vi "Tester.vi"() -> ()   [LabVIEW 2011]
uses:
  <vilib>/Rock Robotics/SystemInterfaces/DIO/FPGA_DIOChannel.ctl
  <vilib>/Rock Robotics/SystemInterfaces/Typedef/FPGA_TypedefDigitalModule.ctl
  <vilib>/Rock Robotics/SystemInterfaces/AI/FPGA_AIChannel.ctl
  <vilib>/Rock Robotics/SystemInterfaces/Typedef/FPGA_TypedefAnalogModule.ctl
  <vilib>/Rock Robotics/SystemInterfaces/DIO/FPGA_DIOPWMChannel.ctl
  <vilib>/Rock Robotics/SystemInterfaces/DIO/FPGA_DIORelayChannel.ctl
  <vilib>/Rock Robotics/WPI/Solenoid/WPI_SolenoidChannel.ctl
  <vilib>/Rock Robotics/SystemInterfaces/Typedef/FPGA_TypedefSolenoidModule.ctl
  <vilib>/Rock Robotics/WPI/Joystick/WPI_JoystickDeviceEnum.ctl
  <vilib>/Rock Robotics/WPI/Solenoid/WPI_SolenoidValue.ctl
  <vilib>/Rock Robotics/WPI/Relay/WPI_RelayValue.ctl
  <vilib>/Rock Robotics/WPI/MotorControl/WPI_MotorControlOpen Jaguar.vi
  <vilib>/Rock Robotics/WPI/Solenoid/WPI_SolenoidOpenSingle.vi
  <vilib>/Rock Robotics/WPI/Solenoid/Deprecated/WPI_SolenoidGetBool.vi
  <vilib>/Rock Robotics/WPI/Solenoid/WPI_SolenoidSetEnum.vi
panel:
  out "Boolean 12":bool
  out "Boolean 11":bool
  out "Boolean 10":bool
  out "Boolean 9":bool
  out "Boolean 8":bool
  out "Boolean 7":bool
  out "Boolean 6":bool
  out "Boolean 5":bool
  out "Boolean 4":bool
  out "Boolean 3":bool
  out "Boolean 2":bool
  out "Boolean":bool
  out "Axis 6":u8
  out "Axis 5":u8
  out "Axis 4":u8
  out "Axis 3 (Throttle)":u8
  out "Axis 2 (Y)":u8
  out "Axis 1 (X)":u8
  in  "Solenoid 8":bool
  in  "Solenoid 7":bool
  in  "Solenoid 6":bool
  in  "Solenoid 5":bool
  in  "Solenoid 4":bool
  in  "Solenoid 3":bool
  in  "Solenoid 2":bool
  in  "Solenoid 1":bool
  in  "Relay 8":bool
  in  "Relay 7":bool
  in  "Relay 6":bool
  in  "Relay 5":bool
  in  "Relay 4":bool
  in  "Relay 3":bool
  in  "Relay 2":bool
  in  "Relay 1":bool
  in  "PWM 10":dbl(knob) scale=-1.0..1.0
  in  "PWM 9":dbl(knob) scale=-1.0..1.0
  in  "PWM 8":dbl(knob) scale=-1.0..1.0
  in  "PWM 7":dbl(knob) scale=-1.0..1.0
  in  "PWM 6":dbl(knob) scale=-1.0..1.0
  in  "PWM 5":dbl(knob) scale=-1.0..1.0
  in  "PWM 4":dbl(knob) scale=-1.0..1.0
  in  "PWM 3":dbl(knob) scale=-1.0..1.0
  in  "PWM 2":dbl(knob) scale=-1.0..1.0
  in  "PWM 1":dbl(knob) scale=-1.0..1.0
  out "Analog 8":dbl
  out "Analog 7":dbl
  out "Analog 6":dbl
  out "Analog 5":dbl
  out "Analog 4":dbl
  out "Analog 3":dbl
  out "Analog 2":dbl
  out "Analog 1":dbl
  out "DIO 14":bool
  out "DIO 13":bool
  out "DIO 12":bool
  out "DIO 11":bool
  out "DIO 10":bool
  out "DIO 9":bool
  out "DIO 8":bool
  out "DIO 7":bool
  out "DIO 6":bool
  out "DIO 5":bool
  out "DIO 4":bool
  out "DIO 3":bool
  out "DIO 2":bool
  out "DIO 1":bool
  # "DIO"
  # "PWM Channels"
  # "Relays"
  # "Solenoids"
  # "Analog"
  # "Joystick"
  # "Buttons"
  # "Axis"
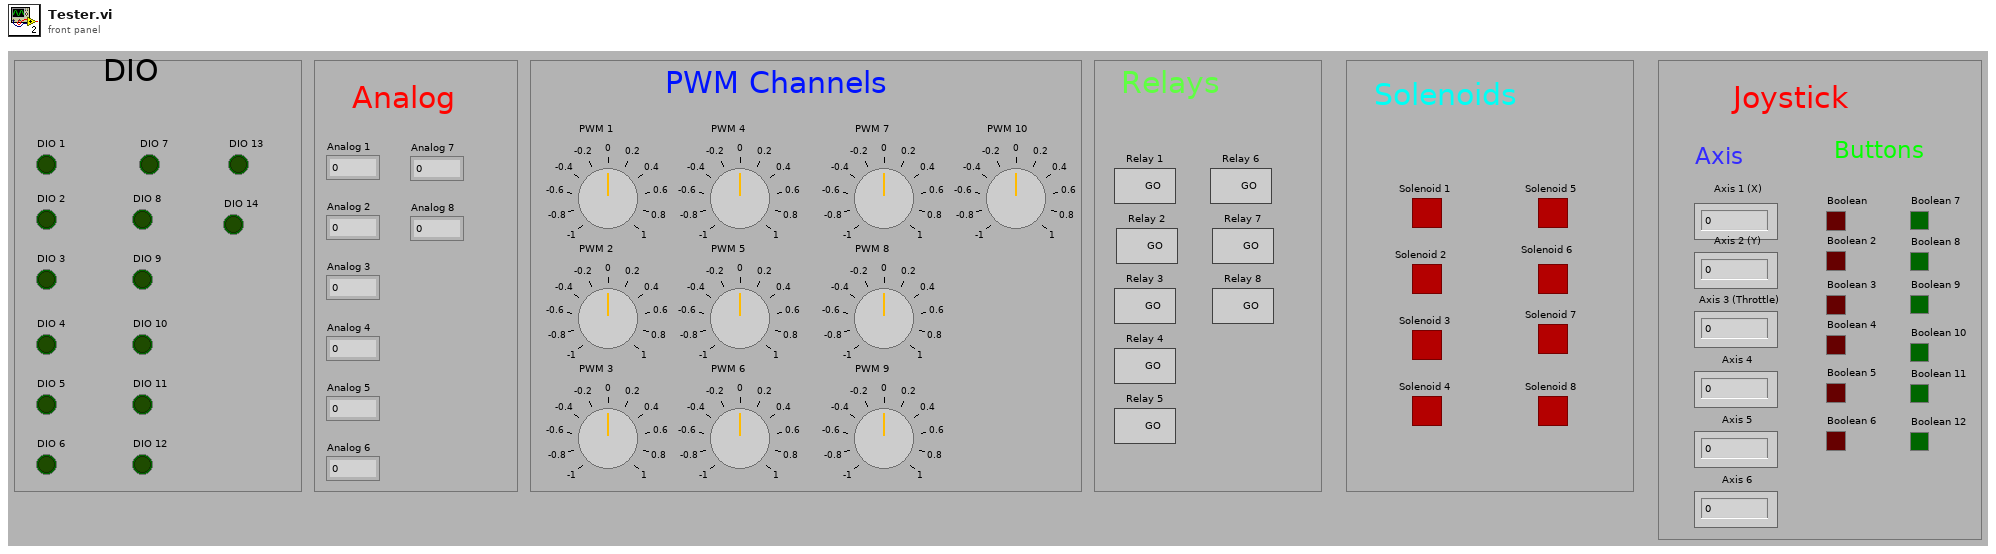
[diagram p1: front panel]
types:
  T1 = typedef "WPI_JoystickDeviceEnum.ctl" = enum16{"USB 1", "USB 2", "USB 3", "USB 4", "Kinect 1", "Kinect 2"}
  T2 = typedef "WPI_SolenoidChannel.ctl" = enum8{"Solenoid 1", "Solenoid 2", "Solenoid 3", "Solenoid 4", "Solenoid 5", "Solenoid 6", "Solenoid 7", "Solenoid 8", "Invalid"}
  T3 = typedef "FPGA_TypedefSolenoidModule.ctl" = enum16{"Solenoid Module 1", "Solenoid Module 2"}
  T4 = typedef "FPGA_DIORelayChannel.ctl" = enum8{"Relay 1", "Relay 2", "Relay 3", "Relay 4", "Relay 5", "Relay 6", "Relay 7", "Relay 8", "Invalid"}
  T5 = typedef "FPGA_TypedefDigitalModule.ctl" = enum16{"Digital Module 1", "Digital Module 2"}
  T6 = typedef "FPGA_DIOPWMChannel.ctl" = enum8{"PWM 1", "PWM 2", "PWM 3", "PWM 4", "PWM 5", "PWM 6", "PWM 7", "PWM 8", "PWM 9", "PWM 10", "Invalid"}
  T7 = typedef "FPGA_AIChannel.ctl" = enum8{"AI 1", "AI 2", "AI 3", "AI 4", "AI 5", "AI 6", "AI 7", "AI 8", "Invalid"}
  T8 = typedef "FPGA_TypedefAnalogModule.ctl" = enum16{"Analog Module 1", "Analog Module 2"}
  T9 = typedef "FPGA_DIOChannel.ctl" = enum8{"DIO 1", "DIO 2", "DIO 3", "DIO 4", "DIO 5", "DIO 6", "DIO 7", "DIO 8", "DIO 9", "DIO 10", "DIO 11", "DIO 12", "DIO 13", "DIO 14", "Invalid"}
  T10 = typedef "WPI_MotorControlDeviceRef.ctl" = cluster{"DeviceStatus":errorcluster, "Type":enum16{"PWM", "CAN"}, "PWM":cluster{"Digital Module":T5, "PWM Channel":T6, "DeadBand":T11}, "CAN":cluster{"Device Number":u8, "Control Mode":T12, "Semaphore":T13, "Max Vout":dbl}, "Invert":bool, "TransformRef":T14, "InvTransformRef":T14}
  T11 = typedef "WPI_PWMDeadband.ctl" = cluster{"Name":string, "maxPositivePwm":i32, "minPositivePwm":i32, "centerPwm":i32, "maxNegativePwm":i32, "minNegativePwm":i32, "angularRange":u16}
  T12 = typedef "WPI_CANJaguar_ControlMode.ctl" = enum8{"Percent VBus", "Current", "Speed", "Position", "Voltage"}
  T13 = typedef "Semaphore RefNum" = refnum<k1>
  T14 = typedef "WPI_PWMTransform_ConPane.ctl" = refnum<vi>
  T15 = typedef "WPI_SolenoidDevRef.ctl" = cluster{"DevStatus":errorcluster, "Solenoid Module":T3, "Forward Solenoid Channel":T2, "Reverse Solenoid Channel":T2}
  T16 = typedef "WPI_DigitalInputDevRef.ctl" = cluster{"DevStatus":errorcluster, "DIO Channel":T9, "Digital Module":T5}
  T17 = typedef "WPI_AnalogChannelDevRef.ctl" = cluster{"DevStatus":errorcluster, "Analog Module":T8, "Analog Channel":T7}
  T18 = typedef "WPI_RelayDevRef.ctl" = cluster{"DevStatus":errorcluster, "Relay Channel":T4, "Digital Module":T5, "Relay Direction":T19}
  T19 = typedef "WPI_RelayDirection.ctl" = enum16{"Both directions", "Forward only", "Reverse only"}
  T20 = typedef "WPI_JoystickDevRef.ctl" = cluster{"Device":T1}
  T21 = typedef "WPI_SolenoidValue.ctl" = enum16{"Off", "On", "Forward", "Reverse"}
  T22 = typedef "WPI_RelayValue.ctl" = enum16{"Off", "On", "Forward", "Reverse"}
  T23 = typedef "WPI_JoystickButtonState.ctl" = cluster{"Button 1":bool, "Button 2":bool, "Button 3":bool, "Button 4":bool, "Button 5":bool, "Button 6":bool, "Button 7":bool, "Button 8":bool, "Button 9":bool, "Button 10":bool, "Button 11":bool, "Button 12":bool}
  T24 = cluster{"axis 1 (x)":dbl, "axis 2 (y)":dbl, "axis 3 (throttle)":dbl, "axis 4":dbl, "axis 5":dbl, "axis 6":dbl}
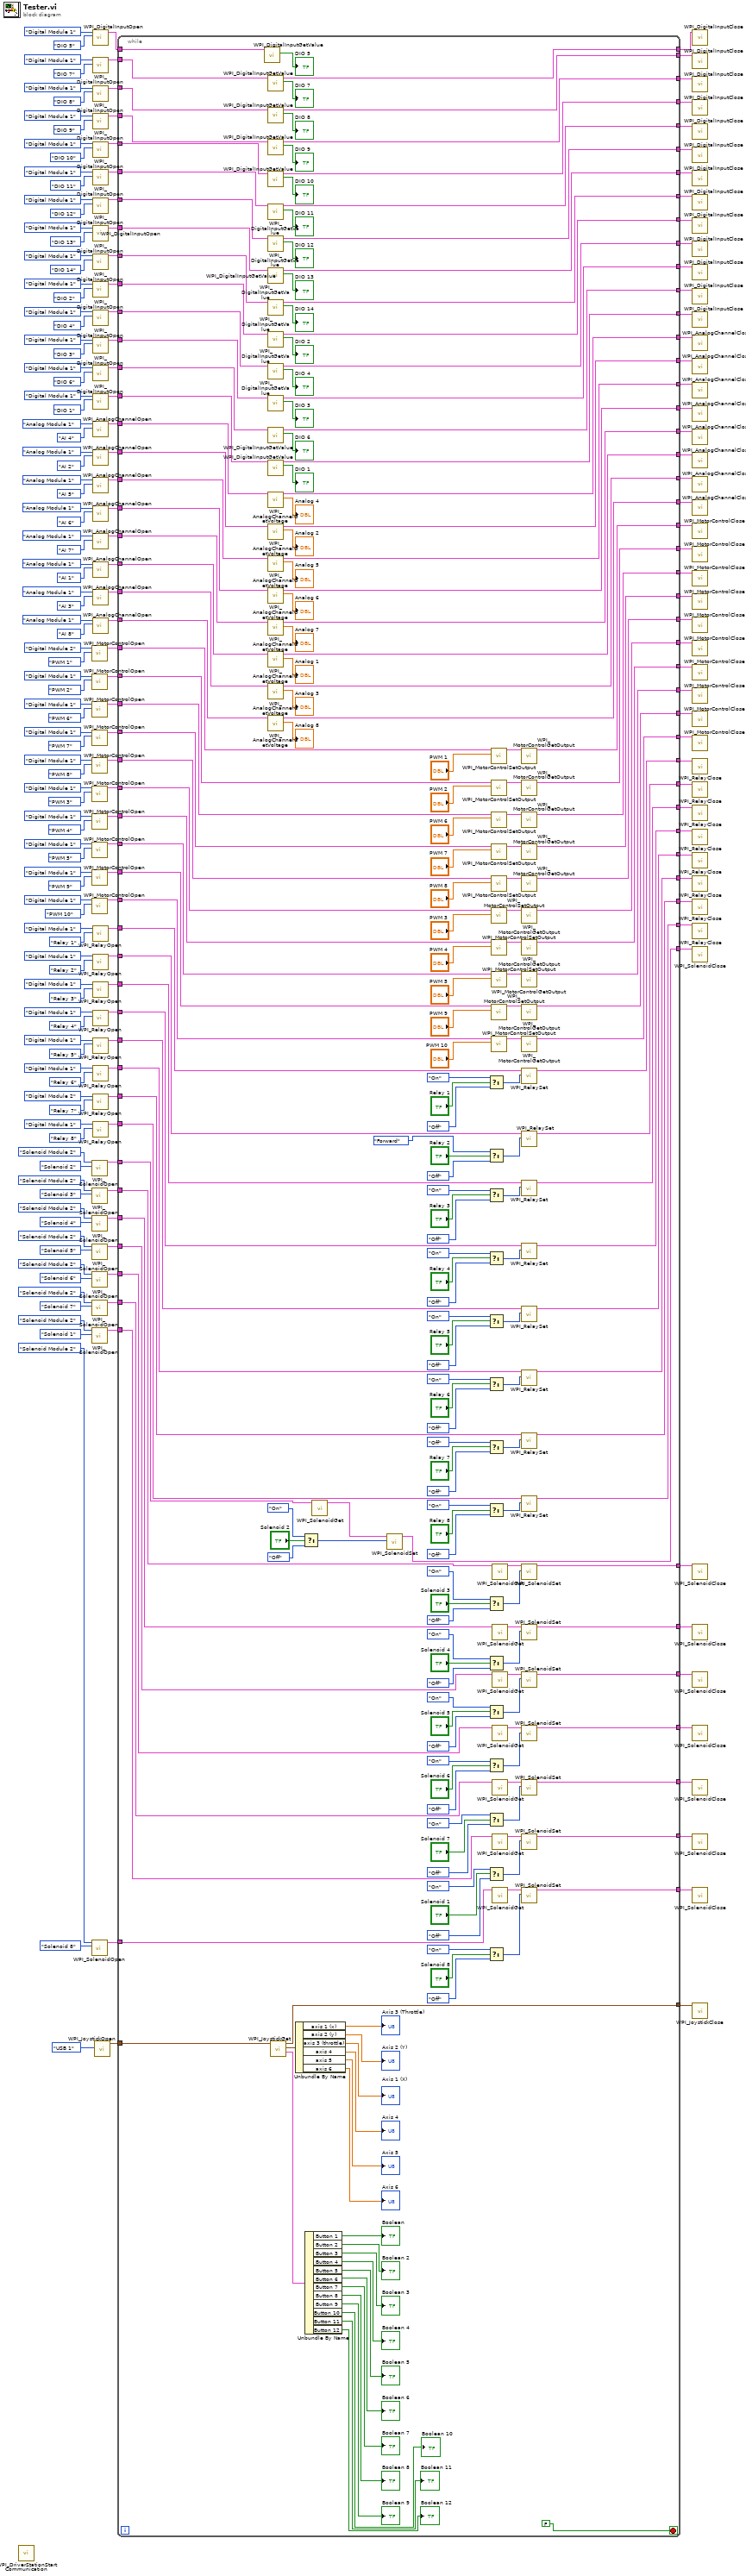
[diagram p0: block diagram]
diagram:
  n1 = call <vilib>:"WPI_DriverStationStart Communication.vi"() -> ()  [unwired: 1 in, 11 out]
  n2 = call-poly <vilib>:"WPI_MotorControlOpen.vi"("PWM Channel"=FPGA_DIOPWMChannel."PWM 1", "Digital Module (Module 1)"=FPGA_TypedefDigitalModule."Digital Module 2" ("DIO Module (Slot 4)")) -> ("MotorControlDeviceRef"=w128:T10)  [unwired: 5 in, 4 out]
  n3 = call-poly <vilib>:"WPI_MotorControlOpen.vi"("PWM Channel"=FPGA_DIOPWMChannel."PWM 2", "Digital Module (Module 1)"=FPGA_TypedefDigitalModule."Digital Module 1" ("DIO Module (Slot 4)")) -> ("MotorControlDeviceRef"=w120:T10)  [unwired: 5 in, 4 out]
  n4 = call-poly <vilib>:"WPI_MotorControlOpen.vi"("PWM Channel"=FPGA_DIOPWMChannel."PWM 6", "Digital Module (Module 1)"=FPGA_TypedefDigitalModule."Digital Module 1" ("DIO Module (Slot 4)")) -> ("MotorControlDeviceRef"=w119:T10)  [unwired: 5 in, 4 out]
  n5 = call-poly <vilib>:"WPI_MotorControlOpen.vi"("PWM Channel"=FPGA_DIOPWMChannel."PWM 7", "Digital Module (Module 1)"=FPGA_TypedefDigitalModule."Digital Module 1" ("DIO Module (Slot 4)")) -> ("MotorControlDeviceRef"=w116:T10)  [unwired: 5 in, 4 out]
  n6 = call-poly <vilib>:"WPI_MotorControlOpen.vi"("PWM Channel"=FPGA_DIOPWMChannel."PWM 8", "Digital Module (Module 1)"=FPGA_TypedefDigitalModule."Digital Module 1" ("DIO Module (Slot 4)")) -> ("MotorControlDeviceRef"=w113:T10)  [unwired: 5 in, 4 out]
  n7 = call-poly <vilib>:"WPI_MotorControlOpen.vi"("PWM Channel"=FPGA_DIOPWMChannel."PWM 3", "Digital Module (Module 1)"=FPGA_TypedefDigitalModule."Digital Module 1" ("DIO Module (Slot 4)")) -> ("MotorControlDeviceRef"=w110:T10)  [unwired: 5 in, 4 out]
  n8 = call-poly <vilib>:"WPI_MotorControlOpen.vi"("PWM Channel"=FPGA_DIOPWMChannel."PWM 4", "Digital Module (Module 1)"=FPGA_TypedefDigitalModule."Digital Module 1" ("DIO Module (Slot 4)")) -> ("MotorControlDeviceRef"=w107:T10)  [unwired: 5 in, 4 out]
  n9 = call-poly <vilib>:"WPI_MotorControlOpen.vi"("PWM Channel"=FPGA_DIOPWMChannel."PWM 5", "Digital Module (Module 1)"=FPGA_TypedefDigitalModule."Digital Module 1" ("DIO Module (Slot 4)")) -> ("MotorControlDeviceRef"=w104:T10)  [unwired: 5 in, 4 out]
  n10 = call-poly <vilib>:"WPI_MotorControlOpen.vi"("PWM Channel"=FPGA_DIOPWMChannel."PWM 9", "Digital Module (Module 1)"=FPGA_TypedefDigitalModule."Digital Module 1" ("DIO Module (Slot 4)")) -> ("MotorControlDeviceRef"=w96:T10)  [unwired: 5 in, 4 out]
  n11 = call-poly <vilib>:"WPI_MotorControlOpen.vi"("PWM Channel"=FPGA_DIOPWMChannel."PWM 10", "Digital Module (Module 1)"=FPGA_TypedefDigitalModule."Digital Module 1" ("DIO Module (Slot 4)")) -> ("MotorControlDeviceRef"=w91:T10)  [unwired: 5 in, 4 out]
  n12 = call-poly <vilib>:"WPI_SolenoidOpen.vi"("Solenoid Channel"=WPI_SolenoidChannel."Solenoid 2", "Solenoid Module (Module 1)"=FPGA_TypedefSolenoidModule."Solenoid Module 2") -> ("SolenoidDevRef"=w61:T15)  [unwired: 8 in, 1 out]
  n13 = call-poly <vilib>:"WPI_SolenoidOpen.vi"("Solenoid Channel"=WPI_SolenoidChannel."Solenoid 3", "Solenoid Module (Module 1)"=FPGA_TypedefSolenoidModule."Solenoid Module 2") -> ("SolenoidDevRef"=w60:T15)  [unwired: 8 in, 1 out]
  n14 = call-poly <vilib>:"WPI_SolenoidOpen.vi"("Solenoid Channel"=WPI_SolenoidChannel."Solenoid 4", "Solenoid Module (Module 1)"=FPGA_TypedefSolenoidModule."Solenoid Module 2") -> ("SolenoidDevRef"=w59:T15)  [unwired: 8 in, 1 out]
  n15 = call-poly <vilib>:"WPI_SolenoidOpen.vi"("Solenoid Channel"=WPI_SolenoidChannel."Solenoid 5", "Solenoid Module (Module 1)"=FPGA_TypedefSolenoidModule."Solenoid Module 2") -> ("SolenoidDevRef"=w58:T15)  [unwired: 8 in, 1 out]
  n16 = call-poly <vilib>:"WPI_SolenoidOpen.vi"("Solenoid Channel"=WPI_SolenoidChannel."Solenoid 6", "Solenoid Module (Module 1)"=FPGA_TypedefSolenoidModule."Solenoid Module 2") -> ("SolenoidDevRef"=w57:T15)  [unwired: 8 in, 1 out]
  n17 = call-poly <vilib>:"WPI_SolenoidOpen.vi"("Solenoid Channel"=WPI_SolenoidChannel."Solenoid 7", "Solenoid Module (Module 1)"=FPGA_TypedefSolenoidModule."Solenoid Module 2") -> ("SolenoidDevRef"=w56:T15)  [unwired: 8 in, 1 out]
  n18 = call-poly <vilib>:"WPI_SolenoidOpen.vi"("Solenoid Channel"=WPI_SolenoidChannel."Solenoid 1", "Solenoid Module (Module 1)"=FPGA_TypedefSolenoidModule."Solenoid Module 2") -> ("SolenoidDevRef"=w55:T15)  [unwired: 8 in, 1 out]
  n19 = call-poly <vilib>:"WPI_SolenoidOpen.vi"("Solenoid Channel"=WPI_SolenoidChannel."Solenoid 8", "Solenoid Module (Module 1)"=FPGA_TypedefSolenoidModule."Solenoid Module 2") -> ("SolenoidDevRef"=w54:T15)  [unwired: 8 in, 1 out]
  n20 = call <vilib>:"WPI_DigitalInputOpen.vi"("DIO Channel"=FPGA_DIOChannel."DIO 5", "Digital Module (Module 1)"=FPGA_TypedefDigitalModule."Digital Module 1" ("DIO Module (Slot 4)")) -> ("DigitalInputDevRef"=w194:T16)  [unwired: 1 in, 8 out]
  n21 = call <vilib>:"WPI_DigitalInputOpen.vi"("DIO Channel"=FPGA_DIOChannel."DIO 7", "Digital Module (Module 1)"=FPGA_TypedefDigitalModule."Digital Module 1" ("DIO Module (Slot 4)")) -> ("DigitalInputDevRef"=w175:T16)  [unwired: 1 in, 8 out]
  n22 = call <vilib>:"WPI_DigitalInputOpen.vi"("DIO Channel"=FPGA_DIOChannel."DIO 8", "Digital Module (Module 1)"=FPGA_TypedefDigitalModule."Digital Module 1" ("DIO Module (Slot 4)")) -> ("DigitalInputDevRef"=w174:T16)  [unwired: 1 in, 8 out]
  n23 = call <vilib>:"WPI_DigitalInputOpen.vi"("DIO Channel"=FPGA_DIOChannel."DIO 9", "Digital Module (Module 1)"=FPGA_TypedefDigitalModule."Digital Module 1" ("DIO Module (Slot 4)")) -> ("DigitalInputDevRef"=w173:T16)  [unwired: 1 in, 8 out]
  n24 = call <vilib>:"WPI_DigitalInputOpen.vi"("DIO Channel"=FPGA_DIOChannel."DIO 10", "Digital Module (Module 1)"=FPGA_TypedefDigitalModule."Digital Module 1" ("DIO Module (Slot 4)")) -> ("DigitalInputDevRef"=w172:T16)  [unwired: 1 in, 8 out]
  n25 = call <vilib>:"WPI_DigitalInputOpen.vi"("DIO Channel"=FPGA_DIOChannel."DIO 11", "Digital Module (Module 1)"=FPGA_TypedefDigitalModule."Digital Module 1" ("DIO Module (Slot 4)")) -> ("DigitalInputDevRef"=w171:T16)  [unwired: 1 in, 8 out]
  n26 = call <vilib>:"WPI_DigitalInputOpen.vi"("DIO Channel"=FPGA_DIOChannel."DIO 12", "Digital Module (Module 1)"=FPGA_TypedefDigitalModule."Digital Module 1" ("DIO Module (Slot 4)")) -> ("DigitalInputDevRef"=w170:T16)  [unwired: 1 in, 8 out]
  n27 = call <vilib>:"WPI_DigitalInputOpen.vi"("DIO Channel"=FPGA_DIOChannel."DIO 13", "Digital Module (Module 1)"=FPGA_TypedefDigitalModule."Digital Module 1" ("DIO Module (Slot 4)")) -> ("DigitalInputDevRef"=w169:T16)  [unwired: 1 in, 8 out]
  n28 = call <vilib>:"WPI_DigitalInputOpen.vi"("DIO Channel"=FPGA_DIOChannel."DIO 14", "Digital Module (Module 1)"=FPGA_TypedefDigitalModule."Digital Module 1" ("DIO Module (Slot 4)")) -> ("DigitalInputDevRef"=w168:T16)  [unwired: 1 in, 8 out]
  n29 = call <vilib>:"WPI_DigitalInputOpen.vi"("DIO Channel"=FPGA_DIOChannel."DIO 2", "Digital Module (Module 1)"=FPGA_TypedefDigitalModule."Digital Module 1" ("DIO Module (Slot 4)")) -> ("DigitalInputDevRef"=w167:T16)  [unwired: 1 in, 8 out]
  n30 = call <vilib>:"WPI_DigitalInputOpen.vi"("DIO Channel"=FPGA_DIOChannel."DIO 4", "Digital Module (Module 1)"=FPGA_TypedefDigitalModule."Digital Module 1" ("DIO Module (Slot 4)")) -> ("DigitalInputDevRef"=w164:T16)  [unwired: 1 in, 8 out]
  n31 = call <vilib>:"WPI_DigitalInputOpen.vi"("DIO Channel"=FPGA_DIOChannel."DIO 3", "Digital Module (Module 1)"=FPGA_TypedefDigitalModule."Digital Module 1" ("DIO Module (Slot 4)")) -> ("DigitalInputDevRef"=w161:T16)  [unwired: 1 in, 8 out]
  n32 = call <vilib>:"WPI_DigitalInputOpen.vi"("DIO Channel"=FPGA_DIOChannel."DIO 6", "Digital Module (Module 1)"=FPGA_TypedefDigitalModule."Digital Module 1" ("DIO Module (Slot 4)")) -> ("DigitalInputDevRef"=w158:T16)  [unwired: 1 in, 8 out]
  n33 = call <vilib>:"WPI_DigitalInputOpen.vi"("DIO Channel"=FPGA_DIOChannel."DIO 1", "Digital Module (Module 1)"=FPGA_TypedefDigitalModule."Digital Module 1" ("DIO Module (Slot 4)")) -> ("DigitalInputDevRef"=w155:T16)  [unwired: 1 in, 8 out]
  n34 = call <vilib>:"WPI_AnalogChannelOpen.vi"("Analog Channel"=FPGA_AIChannel."AI 4", "Analog Module (Module 1)"=FPGA_TypedefAnalogModule."Analog Module 1" ("Analog Module (Slot 1)")) -> ("AIDeviceRef"=w136:T17)  [unwired: 1 in, 8 out]
  n35 = call <vilib>:"WPI_AnalogChannelOpen.vi"("Analog Channel"=FPGA_AIChannel."AI 2", "Analog Module (Module 1)"=FPGA_TypedefAnalogModule."Analog Module 1" ("Analog Module (Slot 1)")) -> ("AIDeviceRef"=w135:T17)  [unwired: 1 in, 8 out]
  n36 = call <vilib>:"WPI_AnalogChannelOpen.vi"("Analog Channel"=FPGA_AIChannel."AI 5", "Analog Module (Module 1)"=FPGA_TypedefAnalogModule."Analog Module 1" ("Analog Module (Slot 1)")) -> ("AIDeviceRef"=w134:T17)  [unwired: 1 in, 8 out]
  n37 = call <vilib>:"WPI_AnalogChannelOpen.vi"("Analog Channel"=FPGA_AIChannel."AI 6", "Analog Module (Module 1)"=FPGA_TypedefAnalogModule."Analog Module 1" ("Analog Module (Slot 1)")) -> ("AIDeviceRef"=w133:T17)  [unwired: 1 in, 8 out]
  n38 = call <vilib>:"WPI_AnalogChannelOpen.vi"("Analog Channel"=FPGA_AIChannel."AI 7", "Analog Module (Module 1)"=FPGA_TypedefAnalogModule."Analog Module 1" ("Analog Module (Slot 1)")) -> ("AIDeviceRef"=w132:T17)  [unwired: 1 in, 8 out]
  n39 = call <vilib>:"WPI_AnalogChannelOpen.vi"("Analog Channel"=FPGA_AIChannel."AI 1", "Analog Module (Module 1)"=FPGA_TypedefAnalogModule."Analog Module 1" ("Analog Module (Slot 1)")) -> ("AIDeviceRef"=w131:T17)  [unwired: 1 in, 8 out]
  n40 = call <vilib>:"WPI_AnalogChannelOpen.vi"("Analog Channel"=FPGA_AIChannel."AI 3", "Analog Module (Module 1)"=FPGA_TypedefAnalogModule."Analog Module 1" ("Analog Module (Slot 1)")) -> ("AIDeviceRef"=w130:T17)  [unwired: 1 in, 8 out]
  n41 = call <vilib>:"WPI_AnalogChannelOpen.vi"("Analog Channel"=FPGA_AIChannel."AI 8", "Analog Module (Module 1)"=FPGA_TypedefAnalogModule."Analog Module 1" ("Analog Module (Slot 1)")) -> ("AIDeviceRef"=w129:T17)  [unwired: 1 in, 8 out]
  n42 = call <vilib>:"WPI_RelayOpen.vi"("Relay Channel"=FPGA_DIORelayChannel."Relay 1", "Digital Module (Module 1)"=FPGA_TypedefDigitalModule."Digital Module 1" ("DIO Module (Slot 4)")) -> ("RelayDevRef"=w86:T18)  [unwired: 2 in, 7 out]
  n43 = call <vilib>:"WPI_RelayOpen.vi"("Relay Channel"=FPGA_DIORelayChannel."Relay 2", "Digital Module (Module 1)"=FPGA_TypedefDigitalModule."Digital Module 1" ("DIO Module (Slot 4)")) -> ("RelayDevRef"=w84:T18)  [unwired: 2 in, 7 out]
  n44 = call <vilib>:"WPI_RelayOpen.vi"("Relay Channel"=FPGA_DIORelayChannel."Relay 3", "Digital Module (Module 1)"=FPGA_TypedefDigitalModule."Digital Module 1" ("DIO Module (Slot 4)")) -> ("RelayDevRef"=w83:T18)  [unwired: 2 in, 7 out]
  n45 = call <vilib>:"WPI_RelayOpen.vi"("Relay Channel"=FPGA_DIORelayChannel."Relay 4", "Digital Module (Module 1)"=FPGA_TypedefDigitalModule."Digital Module 1" ("DIO Module (Slot 4)")) -> ("RelayDevRef"=w82:T18)  [unwired: 2 in, 7 out]
  n46 = call <vilib>:"WPI_RelayOpen.vi"("Relay Channel"=FPGA_DIORelayChannel."Relay 5", "Digital Module (Module 1)"=FPGA_TypedefDigitalModule."Digital Module 1" ("DIO Module (Slot 4)")) -> ("RelayDevRef"=w81:T18)  [unwired: 2 in, 7 out]
  n47 = call <vilib>:"WPI_RelayOpen.vi"("Relay Channel"=FPGA_DIORelayChannel."Relay 6", "Digital Module (Module 1)"=FPGA_TypedefDigitalModule."Digital Module 1" ("DIO Module (Slot 4)")) -> ("RelayDevRef"=w80:T18)  [unwired: 2 in, 7 out]
  n48 = call <vilib>:"WPI_RelayOpen.vi"("Relay Channel"=FPGA_DIORelayChannel."Relay 7", "Digital Module (Module 1)"=FPGA_TypedefDigitalModule."Digital Module 2" ("DIO Module (Slot 4)")) -> ("RelayDevRef"=w79:T18)  [unwired: 2 in, 7 out]
  n49 = call <vilib>:"WPI_RelayOpen.vi"("Relay Channel"=FPGA_DIORelayChannel."Relay 8", "Digital Module (Module 1)"=FPGA_TypedefDigitalModule."Digital Module 1" ("DIO Module (Slot 4)")) -> ("RelayDevRef"=w78:T18)  [unwired: 2 in, 7 out]
  n50 = call <vilib>:"WPI_JoystickOpen.vi"("JoystickDevice"=WPI_JoystickDeviceEnum."USB 1") -> ("JoystickDevRef"=w3:T20)  [unwired: 10 in]
  n51 = while {
    tunnel: w194 -> [w425]
    tunnel: w175 -> [w424]
    tunnel: w174 -> [w423]
    tunnel: w173 -> [w422]
    tunnel: w172 -> [w421]
    tunnel: w171 -> [w420]
    tunnel: w170 -> [w419]
    tunnel: w169 -> [w418]
    tunnel: w168 -> [w417]
    tunnel: w167 -> [w416]
    tunnel: w164 -> [w415]
    tunnel: w161 -> [w414]
    tunnel: w158 -> [w413]
    tunnel: w155 -> [w412]
    tunnel: w136 -> [w411]
    tunnel: w135 -> [w410]
    tunnel: w134 -> [w409]
    tunnel: w133 -> [w408]
    tunnel: w132 -> [w407]
    tunnel: w131 -> [w406]
    tunnel: w130 -> [w405]
    tunnel: w129 -> [w404]
    tunnel: w128 -> [w381]
    tunnel: [w379] -> w127
    tunnel: w120 -> [w371]
    tunnel: w119 -> [w370]
    tunnel: w116 -> [w369]
    tunnel: w113 -> [w368]
    tunnel: w110 -> [w367]
    tunnel: w107 -> [w366]
    tunnel: w104 -> [w365]
    tunnel: [w364] -> w103
    tunnel: [w363] -> w102
    tunnel: [w362] -> w101
    tunnel: [w361] -> w100
    tunnel: [w360] -> w99
    tunnel: [w359] -> w98
    tunnel: [w358] -> w97
    tunnel: w96 -> [w347]
    tunnel: w91 -> [w345]
    tunnel: [w343] -> w90
    tunnel: [w342] -> w89
    tunnel: w86 -> [w341]
    tunnel: [w340] -> w85
    tunnel: w84 -> [w339]
    tunnel: w83 -> [w338]
    tunnel: w82 -> [w337]
    tunnel: w81 -> [w336]
    tunnel: w80 -> [w335]
    tunnel: w79 -> [w334]
    tunnel: w78 -> [w333]
    tunnel: w61 -> [w332]
    tunnel: w60 -> [w331]
    tunnel: w59 -> [w330]
    tunnel: w58 -> [w329]
    tunnel: w57 -> [w328]
    tunnel: w56 -> [w327]
    tunnel: w55 -> [w326]
    tunnel: w54 -> [w325]
    tunnel: [w296] -> w53
    tunnel: [w295] -> w52
    tunnel: [w294] -> w51
    tunnel: [w293] -> w50
    tunnel: [w292] -> w49
    tunnel: [w291] -> w48
    tunnel: [w290] -> w47
    tunnel: [w289] -> w46
    tunnel: [w288] -> w45
    tunnel: [w287] -> w44
    tunnel: [w286] -> w43
    tunnel: [w285] -> w42
    tunnel: [w284] -> w41
    tunnel: [w283] -> w40
    tunnel: [w278] -> w39
    tunnel: [w269] -> w38
    tunnel: [w268] -> w37
    tunnel: [w267] -> w36
    tunnel: [w266] -> w35
    tunnel: [w265] -> w34
    tunnel: [w264] -> w33
    tunnel: [w263] -> w32
    tunnel: [w262] -> w31
    tunnel: [w261] -> w30
    tunnel: [w260] -> w29
    tunnel: [w259] -> w28
    tunnel: [w258] -> w27
    tunnel: [w257] -> w26
    tunnel: [w256] -> w25
    tunnel: [w255] -> w24
    tunnel: [w254] -> w23
    tunnel: [w253] -> w22
    tunnel: [w252] -> w21
    tunnel: [w251] -> w20
    tunnel: [w250] -> w19
    tunnel: [w249] -> w18
    tunnel: w3 -> [w216]
    tunnel: [w215] -> w2
    stop <- FALSE stop-if-true
    n52 = call <vilib>:"WPI_DigitalInputGetValue.vi"("DigitalInputDevRef"=w425) -> ("Value"=→"DIO 5":bool)  [unwired: 1 in, 9 out]
    n53 = call <vilib>:"WPI_DigitalInputGetValue.vi"("DigitalInputDevRef"=w424) -> ("Value"=→"DIO 7":bool, "DigitalInputDevRef"=w258:T16)  [unwired: 1 in, 8 out]
    n54 = call <vilib>:"WPI_DigitalInputGetValue.vi"("DigitalInputDevRef"=w423) -> ("Value"=→"DIO 8":bool, "DigitalInputDevRef"=w259:T16)  [unwired: 1 in, 8 out]
    n55 = call <vilib>:"WPI_DigitalInputGetValue.vi"("DigitalInputDevRef"=w422) -> ("Value"=→"DIO 9":bool, "DigitalInputDevRef"=w260:T16)  [unwired: 1 in, 8 out]
    n56 = call <vilib>:"WPI_DigitalInputGetValue.vi"("DigitalInputDevRef"=w421) -> ("Value"=→"DIO 10":bool, "DigitalInputDevRef"=w263:T16)  [unwired: 1 in, 8 out]
    n57 = call <vilib>:"WPI_DigitalInputGetValue.vi"("DigitalInputDevRef"=w420) -> ("Value"=→"DIO 11":bool, "DigitalInputDevRef"=w261:T16)  [unwired: 1 in, 8 out]
    n58 = call <vilib>:"WPI_DigitalInputGetValue.vi"("DigitalInputDevRef"=w419) -> ("Value"=→"DIO 12":bool, "DigitalInputDevRef"=w262:T16)  [unwired: 1 in, 8 out]
    n59 = call <vilib>:"WPI_DigitalInputGetValue.vi"("DigitalInputDevRef"=w418) -> ("Value"=→"DIO 13":bool, "DigitalInputDevRef"=w257:T16)  [unwired: 1 in, 8 out]
    n60 = call <vilib>:"WPI_DigitalInputGetValue.vi"("DigitalInputDevRef"=w417) -> ("Value"=→"DIO 14":bool, "DigitalInputDevRef"=w264:T16)  [unwired: 1 in, 8 out]
    n61 = call <vilib>:"WPI_DigitalInputGetValue.vi"("DigitalInputDevRef"=w416) -> ("Value"=→"DIO 2":bool, "DigitalInputDevRef"=w265:T16)  [unwired: 1 in, 8 out]
    n62 = call <vilib>:"WPI_DigitalInputGetValue.vi"("DigitalInputDevRef"=w415) -> ("Value"=→"DIO 4":bool, "DigitalInputDevRef"=w266:T16)  [unwired: 1 in, 8 out]
    n63 = call <vilib>:"WPI_DigitalInputGetValue.vi"("DigitalInputDevRef"=w414) -> ("Value"=→"DIO 3":bool, "DigitalInputDevRef"=w267:T16)  [unwired: 1 in, 8 out]
    n64 = call <vilib>:"WPI_DigitalInputGetValue.vi"("DigitalInputDevRef"=w413) -> ("Value"=→"DIO 6":bool, "DigitalInputDevRef"=w268:T16)  [unwired: 1 in, 8 out]
    n65 = call <vilib>:"WPI_DigitalInputGetValue.vi"("DigitalInputDevRef"=w412) -> ("Value"=→"DIO 1":bool, "DigitalInputDevRef"=w269:T16)  [unwired: 1 in, 8 out]
    n66 = call <vilib>:"WPI_AnalogChannelGetVoltage.vi"("AIDeviceRef"=w411) -> ("Voltage"=→"Analog 4":dbl, "AIDeviceRef"=w256:T17)  [unwired: 1 in, 8 out]
    n67 = call <vilib>:"WPI_AnalogChannelGetVoltage.vi"("AIDeviceRef"=w410) -> ("Voltage"=→"Analog 2":dbl, "AIDeviceRef"=w254:T17)  [unwired: 1 in, 8 out]
    n68 = call <vilib>:"WPI_AnalogChannelGetVoltage.vi"("AIDeviceRef"=w409) -> ("Voltage"=→"Analog 5":dbl, "AIDeviceRef"=w253:T17)  [unwired: 1 in, 8 out]
    n69 = call <vilib>:"WPI_AnalogChannelGetVoltage.vi"("AIDeviceRef"=w408) -> ("Voltage"=→"Analog 6":dbl, "AIDeviceRef"=w252:T17)  [unwired: 1 in, 8 out]
    n70 = call <vilib>:"WPI_AnalogChannelGetVoltage.vi"("AIDeviceRef"=w407) -> ("Voltage"=→"Analog 7":dbl, "AIDeviceRef"=w251:T17)  [unwired: 1 in, 8 out]
    n71 = call <vilib>:"WPI_AnalogChannelGetVoltage.vi"("AIDeviceRef"=w406) -> ("Voltage"=→"Analog 1":dbl, "AIDeviceRef"=w250:T17)  [unwired: 1 in, 8 out]
    n72 = call <vilib>:"WPI_AnalogChannelGetVoltage.vi"("AIDeviceRef"=w405) -> ("Voltage"=→"Analog 3":dbl, "AIDeviceRef"=w249:T17)  [unwired: 1 in, 8 out]
    n73 = call <vilib>:"WPI_AnalogChannelGetVoltage.vi"("AIDeviceRef"=w404) -> ("Voltage"=→"Analog 8":dbl, "AIDeviceRef"=w255:T17)  [unwired: 1 in, 8 out]
    n74 = call <vilib>:"WPI_JoystickGet.vi"("JoystickDevRef"=w216) -> ("Buttons"=w213:T23, "Axes"=w214:T24, "JoystickDevRef"=w215:T20)  [unwired: 4 in]
    n75 = Unbundle By Name(w214) -> ("axis 1 (x)"=→"Axis 3 (Throttle)":dbl, "axis 2 (y)"=→"Axis 2 (Y)":dbl, "axis 3 (throttle)"=→"Axis 1 (X)":dbl, "axis 4"=→"Axis 4":dbl, "axis 5"=→"Axis 5":dbl, "axis 6"=→"Axis 6":dbl)
    n76 = Select(t=WPI_SolenoidValue."On" ("Value"), s="Solenoid 2", f=WPI_SolenoidValue."Off" ("Value")) -> (s? t:f=w234:T21)
    n77 = Unbundle By Name(w213) -> ("Button 1"=→"Boolean":bool, "Button 2"=→"Boolean 2":bool, "Button 3"=→"Boolean 3":bool, "Button 4"=→"Boolean 4":bool, "Button 5"=→"Boolean 5":bool, "Button 6"=→"Boolean 6":bool, "Button 7"=→"Boolean 7":bool, "Button 8"=→"Boolean 8":bool, "Button 9"=→"Boolean 9":bool, "Button 10"=→"Boolean 10":bool, "Button 11"=→"Boolean 11":bool, "Button 12"=→"Boolean 12":bool)
    n78 = call-poly <vilib>:"WPI_SolenoidGet.vi"("SolenoidDevRef"=w332) -> ("SolenoidDevRef"=w279:T15)  [unwired: 8 in, 2 out]
    n79 = call-poly <vilib>:"WPI_SolenoidSet.vi"("Value"=w234, "SolenoidDevRef"=w279) -> ("SolenoidDevRef"=w288:T15)  [unwired: 8 in, 1 out]
    n80 = Select(t=WPI_RelayValue."On" ("RelayValue"), s="Relay 1", f=WPI_RelayValue."Off" ("RelayValue")) -> (s? t:f=w297:T22)
    n81 = Select(t=WPI_RelayValue."Forward" ("RelayValue"), s="Relay 2", f=WPI_RelayValue."Off" ("RelayValue")) -> (s? t:f=w300:T22)
    n82 = Select(t=WPI_RelayValue."On" ("RelayValue"), s="Relay 3", f=WPI_RelayValue."Off" ("RelayValue")) -> (s? t:f=w309:T22)
    n83 = Select(t=WPI_RelayValue."On" ("RelayValue"), s="Relay 4", f=WPI_RelayValue."Off" ("RelayValue")) -> (s? t:f=w303:T22)
    n84 = Select(t=WPI_RelayValue."On" ("RelayValue"), s="Relay 5", f=WPI_RelayValue."Off" ("RelayValue")) -> (s? t:f=w315:T22)
    n85 = Select(t=WPI_RelayValue."On" ("RelayValue"), s="Relay 6", f=WPI_RelayValue."Off" ("RelayValue")) -> (s? t:f=w306:T22)
    n86 = Select(t=WPI_RelayValue."Off" ("RelayValue"), s="Relay 7", f=WPI_RelayValue."Off" ("RelayValue")) -> (s? t:f=w320:T22)
    n87 = Select(t=WPI_RelayValue."On" ("RelayValue"), s="Relay 8", f=WPI_RelayValue."Off" ("RelayValue")) -> (s? t:f=w312:T22)
    n88 = Select(t=WPI_SolenoidValue."On" ("Value"), s="Solenoid 3", f=WPI_SolenoidValue."Off" ("Value")) -> (s? t:f=w237:T21)
    n89 = Select(t=WPI_SolenoidValue."On" ("Value"), s="Solenoid 4", f=WPI_SolenoidValue."Off" ("Value")) -> (s? t:f=w240:T21)
    n90 = Select(t=WPI_SolenoidValue."On" ("Value"), s="Solenoid 5", f=WPI_SolenoidValue."Off" ("Value")) -> (s? t:f=w243:T21)
    n91 = Select(t=WPI_SolenoidValue."On" ("Value"), s="Solenoid 6", f=WPI_SolenoidValue."Off" ("Value")) -> (s? t:f=w246:T21)
    n92 = Select(t=WPI_SolenoidValue."On" ("Value"), s="Solenoid 7", f=WPI_SolenoidValue."Off" ("Value")) -> (s? t:f=w217:T21)
    n93 = Select(t=WPI_SolenoidValue."On" ("Value"), s="Solenoid 1", f=WPI_SolenoidValue."Off" ("Value")) -> (s? t:f=w231:T21)
    n94 = Select(t=WPI_SolenoidValue."On" ("Value"), s="Solenoid 8", f=WPI_SolenoidValue."Off" ("Value")) -> (s? t:f=w228:T21)
    n95 = call <vilib>:"WPI_MotorControlSetOutput.vi"("Output"="PWM 1", "MotorControlDevRef"=w381) -> ("MotorControlDevRef"=w380:T10)  [unwired: 3 in, 6 out]
    n96 = call <vilib>:"WPI_MotorControlSetOutput.vi"("Output"="PWM 2", "MotorControlDevRef"=w371) -> ("MotorControlDevRef"=w378:T10)  [unwired: 3 in, 6 out]
    n97 = call <vilib>:"WPI_MotorControlSetOutput.vi"("Output"="PWM 6", "MotorControlDevRef"=w370) -> ("MotorControlDevRef"=w377:T10)  [unwired: 3 in, 6 out]
    n98 = call <vilib>:"WPI_MotorControlSetOutput.vi"("Output"="PWM 7", "MotorControlDevRef"=w369) -> ("MotorControlDevRef"=w376:T10)  [unwired: 3 in, 6 out]
    n99 = call <vilib>:"WPI_MotorControlSetOutput.vi"("Output"="PWM 8", "MotorControlDevRef"=w368) -> ("MotorControlDevRef"=w375:T10)  [unwired: 3 in, 6 out]
    n100 = call <vilib>:"WPI_MotorControlSetOutput.vi"("Output"="PWM 3", "MotorControlDevRef"=w367) -> ("MotorControlDevRef"=w372:T10)  [unwired: 3 in, 6 out]
    n101 = call <vilib>:"WPI_MotorControlSetOutput.vi"("Output"="PWM 4", "MotorControlDevRef"=w366) -> ("MotorControlDevRef"=w373:T10)  [unwired: 3 in, 6 out]
    n102 = call <vilib>:"WPI_MotorControlSetOutput.vi"("Output"="PWM 5", "MotorControlDevRef"=w365) -> ("MotorControlDevRef"=w374:T10)  [unwired: 3 in, 6 out]
    n103 = call <vilib>:"WPI_MotorControlSetOutput.vi"("Output"="PWM 9", "MotorControlDevRef"=w347) -> ("MotorControlDevRef"=w352:T10)  [unwired: 3 in, 6 out]
    n104 = call <vilib>:"WPI_MotorControlSetOutput.vi"("Output"="PWM 10", "MotorControlDevRef"=w345) -> ("MotorControlDevRef"=w351:T10)  [unwired: 3 in, 6 out]
    n105 = call-poly <vilib>:"WPI_SolenoidGet.vi"("SolenoidDevRef"=w331) -> ("SolenoidDevRef"=w280:T15)  [unwired: 8 in, 2 out]
    n106 = call-poly <vilib>:"WPI_SolenoidGet.vi"("SolenoidDevRef"=w330) -> ("SolenoidDevRef"=w281:T15)  [unwired: 8 in, 2 out]
    n107 = call-poly <vilib>:"WPI_SolenoidGet.vi"("SolenoidDevRef"=w329) -> ("SolenoidDevRef"=w282:T15)  [unwired: 8 in, 2 out]
    n108 = call-poly <vilib>:"WPI_SolenoidGet.vi"("SolenoidDevRef"=w328) -> ("SolenoidDevRef"=w321:T15)  [unwired: 8 in, 2 out]
    n109 = call-poly <vilib>:"WPI_SolenoidGet.vi"("SolenoidDevRef"=w327) -> ("SolenoidDevRef"=w322:T15)  [unwired: 8 in, 2 out]
    n110 = call-poly <vilib>:"WPI_SolenoidGet.vi"("SolenoidDevRef"=w326) -> ("SolenoidDevRef"=w323:T15)  [unwired: 8 in, 2 out]
    n111 = call-poly <vilib>:"WPI_SolenoidGet.vi"("SolenoidDevRef"=w325) -> ("SolenoidDevRef"=w324:T15)  [unwired: 8 in, 2 out]
    n112 = call <vilib>:"WPI_MotorControlGetOutput.vi"("MotorControlDevRef"=w380) -> ("MotorControlDevRef"=w379:T10)  [unwired: 1 in, 9 out]
    n113 = call <vilib>:"WPI_MotorControlGetOutput.vi"("MotorControlDevRef"=w378) -> ("MotorControlDevRef"=w364:T10)  [unwired: 1 in, 9 out]
    n114 = call <vilib>:"WPI_MotorControlGetOutput.vi"("MotorControlDevRef"=w377) -> ("MotorControlDevRef"=w360:T10)  [unwired: 1 in, 9 out]
    n115 = call <vilib>:"WPI_MotorControlGetOutput.vi"("MotorControlDevRef"=w376) -> ("MotorControlDevRef"=w359:T10)  [unwired: 1 in, 9 out]
    n116 = call <vilib>:"WPI_MotorControlGetOutput.vi"("MotorControlDevRef"=w375) -> ("MotorControlDevRef"=w358:T10)  [unwired: 1 in, 9 out]
    n117 = call <vilib>:"WPI_MotorControlGetOutput.vi"("MotorControlDevRef"=w372) -> ("MotorControlDevRef"=w363:T10)  [unwired: 1 in, 9 out]
    n118 = call <vilib>:"WPI_MotorControlGetOutput.vi"("MotorControlDevRef"=w373) -> ("MotorControlDevRef"=w362:T10)  [unwired: 1 in, 9 out]
    n119 = call <vilib>:"WPI_MotorControlGetOutput.vi"("MotorControlDevRef"=w374) -> ("MotorControlDevRef"=w361:T10)  [unwired: 1 in, 9 out]
    n120 = call <vilib>:"WPI_MotorControlGetOutput.vi"("MotorControlDevRef"=w352) -> ("MotorControlDevRef"=w342:T10)  [unwired: 1 in, 9 out]
    n121 = call <vilib>:"WPI_MotorControlGetOutput.vi"("MotorControlDevRef"=w351) -> ("MotorControlDevRef"=w343:T10)  [unwired: 1 in, 9 out]
    n122 = call <vilib>:"WPI_RelaySet.vi"("RelayValue"=w297, "RelayDevRef"=w341) -> ("RelayDevRef"=w340:T18)  [unwired: 1 in, 8 out]
    n123 = call <vilib>:"WPI_RelaySet.vi"("RelayValue"=w300, "RelayDevRef"=w339) -> ("RelayDevRef"=w296:T18)  [unwired: 1 in, 8 out]
    n124 = call <vilib>:"WPI_RelaySet.vi"("RelayValue"=w309, "RelayDevRef"=w338) -> ("RelayDevRef"=w295:T18)  [unwired: 1 in, 8 out]
    n125 = call <vilib>:"WPI_RelaySet.vi"("RelayValue"=w303, "RelayDevRef"=w337) -> ("RelayDevRef"=w294:T18)  [unwired: 1 in, 8 out]
    n126 = call <vilib>:"WPI_RelaySet.vi"("RelayValue"=w315, "RelayDevRef"=w336) -> ("RelayDevRef"=w293:T18)  [unwired: 1 in, 8 out]
    n127 = call <vilib>:"WPI_RelaySet.vi"("RelayValue"=w306, "RelayDevRef"=w335) -> ("RelayDevRef"=w292:T18)  [unwired: 1 in, 8 out]
    n128 = call <vilib>:"WPI_RelaySet.vi"("RelayValue"=w320, "RelayDevRef"=w334) -> ("RelayDevRef"=w291:T18)  [unwired: 1 in, 8 out]
    n129 = call <vilib>:"WPI_RelaySet.vi"("RelayValue"=w312, "RelayDevRef"=w333) -> ("RelayDevRef"=w290:T18)  [unwired: 1 in, 8 out]
    n130 = call-poly <vilib>:"WPI_SolenoidSet.vi"("Value"=w237, "SolenoidDevRef"=w280) -> ("SolenoidDevRef"=w287:T15)  [unwired: 8 in, 1 out]
    n131 = call-poly <vilib>:"WPI_SolenoidSet.vi"("Value"=w240, "SolenoidDevRef"=w281) -> ("SolenoidDevRef"=w286:T15)  [unwired: 8 in, 1 out]
    n132 = call-poly <vilib>:"WPI_SolenoidSet.vi"("Value"=w243, "SolenoidDevRef"=w282) -> ("SolenoidDevRef"=w289:T15)  [unwired: 8 in, 1 out]
    n133 = call-poly <vilib>:"WPI_SolenoidSet.vi"("Value"=w246, "SolenoidDevRef"=w321) -> ("SolenoidDevRef"=w285:T15)  [unwired: 8 in, 1 out]
    n134 = call-poly <vilib>:"WPI_SolenoidSet.vi"("Value"=w217, "SolenoidDevRef"=w322) -> ("SolenoidDevRef"=w284:T15)  [unwired: 8 in, 1 out]
    n135 = call-poly <vilib>:"WPI_SolenoidSet.vi"("Value"=w231, "SolenoidDevRef"=w323) -> ("SolenoidDevRef"=w283:T15)  [unwired: 8 in, 1 out]
    n136 = call-poly <vilib>:"WPI_SolenoidSet.vi"("Value"=w228, "SolenoidDevRef"=w324) -> ("SolenoidDevRef"=w278:T15)  [unwired: 8 in, 1 out]
  }
  n137 = call <vilib>:"WPI_DigitalInputClose.vi"("DigitalInputDevRef"=w27) -> ()  [unwired: 10 in, 1 out]
  n138 = call <vilib>:"WPI_DigitalInputClose.vi"("DigitalInputDevRef"=w28) -> ()  [unwired: 10 in, 1 out]
  n139 = call <vilib>:"WPI_DigitalInputClose.vi"("DigitalInputDevRef"=w29) -> ()  [unwired: 10 in, 1 out]
  n140 = call <vilib>:"WPI_DigitalInputClose.vi"("DigitalInputDevRef"=w32) -> ()  [unwired: 10 in, 1 out]
  n141 = call <vilib>:"WPI_DigitalInputClose.vi"("DigitalInputDevRef"=w30) -> ()  [unwired: 10 in, 1 out]
  n142 = call <vilib>:"WPI_DigitalInputClose.vi"("DigitalInputDevRef"=w31) -> ()  [unwired: 10 in, 1 out]
  n143 = call <vilib>:"WPI_DigitalInputClose.vi"("DigitalInputDevRef"=w26) -> ()  [unwired: 10 in, 1 out]
  n144 = call <vilib>:"WPI_DigitalInputClose.vi"("DigitalInputDevRef"=w33) -> ()  [unwired: 10 in, 1 out]
  n145 = call <vilib>:"WPI_DigitalInputClose.vi"("DigitalInputDevRef"=w34) -> ()  [unwired: 10 in, 1 out]
  n146 = call <vilib>:"WPI_DigitalInputClose.vi"("DigitalInputDevRef"=w35) -> ()  [unwired: 10 in, 1 out]
  n147 = call <vilib>:"WPI_DigitalInputClose.vi"("DigitalInputDevRef"=w36) -> ()  [unwired: 10 in, 1 out]
  n148 = call <vilib>:"WPI_DigitalInputClose.vi"("DigitalInputDevRef"=w37) -> ()  [unwired: 10 in, 1 out]
  n149 = call <vilib>:"WPI_DigitalInputClose.vi"("DigitalInputDevRef"=w38) -> ()  [unwired: 10 in, 1 out]
  n150 = call <vilib>:"WPI_AnalogChannelClose.vi"("AIDeviceRef"=w25) -> ()  [unwired: 10 in, 1 out]
  n151 = call <vilib>:"WPI_AnalogChannelClose.vi"("AIDeviceRef"=w23) -> ()  [unwired: 10 in, 1 out]
  n152 = call <vilib>:"WPI_AnalogChannelClose.vi"("AIDeviceRef"=w22) -> ()  [unwired: 10 in, 1 out]
  n153 = call <vilib>:"WPI_AnalogChannelClose.vi"("AIDeviceRef"=w21) -> ()  [unwired: 10 in, 1 out]
  n154 = call <vilib>:"WPI_AnalogChannelClose.vi"("AIDeviceRef"=w20) -> ()  [unwired: 10 in, 1 out]
  n155 = call <vilib>:"WPI_AnalogChannelClose.vi"("AIDeviceRef"=w19) -> ()  [unwired: 10 in, 1 out]
  n156 = call <vilib>:"WPI_AnalogChannelClose.vi"("AIDeviceRef"=w18) -> ()  [unwired: 10 in, 1 out]
  n157 = call <vilib>:"WPI_AnalogChannelClose.vi"("AIDeviceRef"=w24) -> ()  [unwired: 10 in, 1 out]
  n158 = call <vilib>:"WPI_MotorControlClose.vi"("MotorControlDevRef"=w127) -> ()  [unwired: 1 in, 10 out]
  n159 = call <vilib>:"WPI_MotorControlClose.vi"("MotorControlDevRef"=w103) -> ()  [unwired: 1 in, 10 out]
  n160 = call <vilib>:"WPI_MotorControlClose.vi"("MotorControlDevRef"=w99) -> ()  [unwired: 1 in, 10 out]
  n161 = call <vilib>:"WPI_MotorControlClose.vi"("MotorControlDevRef"=w98) -> ()  [unwired: 1 in, 10 out]
  n162 = call <vilib>:"WPI_MotorControlClose.vi"("MotorControlDevRef"=w97) -> ()  [unwired: 1 in, 10 out]
  n163 = call <vilib>:"WPI_MotorControlClose.vi"("MotorControlDevRef"=w102) -> ()  [unwired: 1 in, 10 out]
  n164 = call <vilib>:"WPI_MotorControlClose.vi"("MotorControlDevRef"=w101) -> ()  [unwired: 1 in, 10 out]
  n165 = call <vilib>:"WPI_MotorControlClose.vi"("MotorControlDevRef"=w100) -> ()  [unwired: 1 in, 10 out]
  n166 = call <vilib>:"WPI_MotorControlClose.vi"("MotorControlDevRef"=w89) -> ()  [unwired: 1 in, 10 out]
  n167 = call <vilib>:"WPI_MotorControlClose.vi"("MotorControlDevRef"=w90) -> ()  [unwired: 1 in, 10 out]
  n168 = call <vilib>:"WPI_RelayClose.vi"("RelayDevRef"=w85) -> ()  [unwired: 1 in, 10 out]
  n169 = call <vilib>:"WPI_RelayClose.vi"("RelayDevRef"=w53) -> ()  [unwired: 10 in, 1 out]
  n170 = call <vilib>:"WPI_RelayClose.vi"("RelayDevRef"=w52) -> ()  [unwired: 10 in, 1 out]
  n171 = call <vilib>:"WPI_RelayClose.vi"("RelayDevRef"=w51) -> ()  [unwired: 10 in, 1 out]
  n172 = call <vilib>:"WPI_RelayClose.vi"("RelayDevRef"=w50) -> ()  [unwired: 10 in, 1 out]
  n173 = call <vilib>:"WPI_RelayClose.vi"("RelayDevRef"=w49) -> ()  [unwired: 10 in, 1 out]
  n174 = call <vilib>:"WPI_RelayClose.vi"("RelayDevRef"=w48) -> ()  [unwired: 10 in, 1 out]
  n175 = call <vilib>:"WPI_RelayClose.vi"("RelayDevRef"=w47) -> ()  [unwired: 10 in, 1 out]
  n176 = call <vilib>:"WPI_SolenoidClose.vi"("SolenoidDevRef"=w45) -> ()  [unwired: 10 in, 1 out]
  n177 = call <vilib>:"WPI_SolenoidClose.vi"("SolenoidDevRef"=w44) -> ()  [unwired: 10 in, 1 out]
  n178 = call <vilib>:"WPI_SolenoidClose.vi"("SolenoidDevRef"=w43) -> ()  [unwired: 10 in, 1 out]
  n179 = call <vilib>:"WPI_SolenoidClose.vi"("SolenoidDevRef"=w46) -> ()  [unwired: 10 in, 1 out]
  n180 = call <vilib>:"WPI_SolenoidClose.vi"("SolenoidDevRef"=w42) -> ()  [unwired: 10 in, 1 out]
  n181 = call <vilib>:"WPI_SolenoidClose.vi"("SolenoidDevRef"=w41) -> ()  [unwired: 10 in, 1 out]
  n182 = call <vilib>:"WPI_SolenoidClose.vi"("SolenoidDevRef"=w40) -> ()  [unwired: 10 in, 1 out]
  n183 = call <vilib>:"WPI_SolenoidClose.vi"("SolenoidDevRef"=w39) -> ()  [unwired: 10 in, 1 out]
  n184 = call <vilib>:"WPI_JoystickClose.vi"("JoystickDevRef"=w2) -> ()  [unwired: 11 in]
